vi "Actor Core.vi"(8 "error in":errorcluster, 11 "User Console":refnum<class "User Console.lvclass">) -> (0 "error out":errorcluster, 3 "Actor out":refnum<class "Actor.lvclass">)   [LabVIEW 2019, in "User Console Actor.lvlib" / "User Console.lvclass"]
doc: "This is Actor Core.vi, the main message handling loop for Actors. An actor usually just sits in this loop and processes messages as they arrive. Any error returned by the message Do.vi call will stop the loop, with error code 43 as the canonical signal to stop with no error sent to caller. Descendants may override that in Handle Error.vi."
uses:
  User Console.lvclass
  <vilib>/ActorFramework/Actor/Actor.lvclass
  <vilib>/ActorFramework/Stop Msg/Stop Msg.lvclass
  C:/Workspace/CLA/Elevator AF/Abstract User Console Actor/Abstract User Console Actor/Abstract User Console.lvclass
  C:/Program Files (x86)/National Instruments/LabVIEW 2019/vi.lib/ActorFramework/Actor/Actor.lvclass
  Abstract User Console Actor/Abstract User Console Actor/Abstract User Console.lvclass
  Elevator Controller Actor/Elevator Control Actor/States -Enum.ctl
  Elevator Controller Actor/Elevator Control Actor/Elevator Controller.lvclass
  Elevator Controller Actor/Elevator Controller Messages/Set State Msg/Set State Msg.lvclass
  Display Console/Display Console/Display Console.lvclass
  Door Buttons.ctl
  Elevator Call.ctl
  Floor Selection.ctl
panel:
  in  "Floor Selection":T1
  in  "Elevator Call":T2
  in  "Emergency Button":bool
  in  "Door Buttons":T3
  # "[Covers: UI1]"
  # "[Covers: UI2]"
  # "[Covers: UI2A] \n[Covers: UI2A1] \n[Covers: UI2A2]"
  # "[Covers: UI2B] \n[Covers: UI2B1] \n[Covers: UI2B2]"
  # "[Covers: UI2C] \n[Covers: UI2C1] \n[Covers: UI2C2] \n[Covers: UI2C3]"
  # "[Covers: UI2D] \n[Covers: UI2D1]"
  # "Fourth Floor"
  # "Third Floor"
  # "Second Floor"
  # "First Floor"
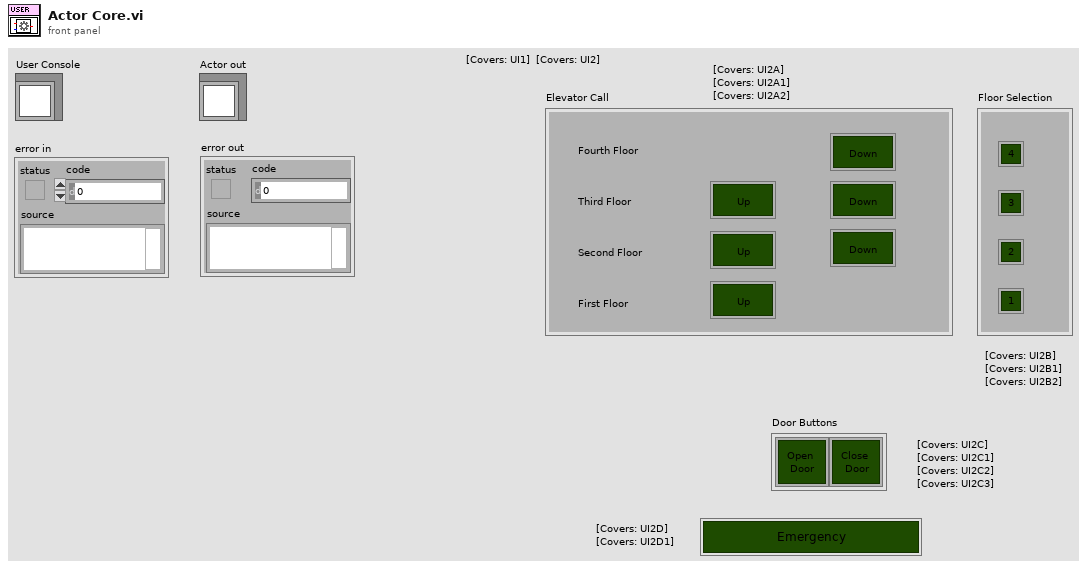
[diagram p1: front panel]
types:
  T1 = typedef "User Console Actor.lvlib/User Console.lvclass/Floor Selection.ctl" = cluster{"Floor4":bool, "Floor 3":bool, "Floor2":bool, "Floor1":bool}
  T2 = typedef "User Console Actor.lvlib/User Console.lvclass/Elevator Call.ctl" = cluster{"Up":bool, "Up 2":bool, "Up 3":bool, "Down":bool, "Down 2":bool, "Down 3":bool}
  T3 = typedef "User Console Actor.lvlib/User Console.lvclass/Door Buttons.ctl" = cluster{"Open Door":bool, "Close Door":bool}
  T4 = typedef "Elevator Controller Actor.lvlib/Elevator Controller.lvclass/States -Enum.ctl" = enum16{"Initial State", "Start and Move State", "Analysis State", "Continue Travel State", "Open and Close Door Sequence", "Stop at Floor", "No Request remaining", "Emergency Call", "Terminate Process"}
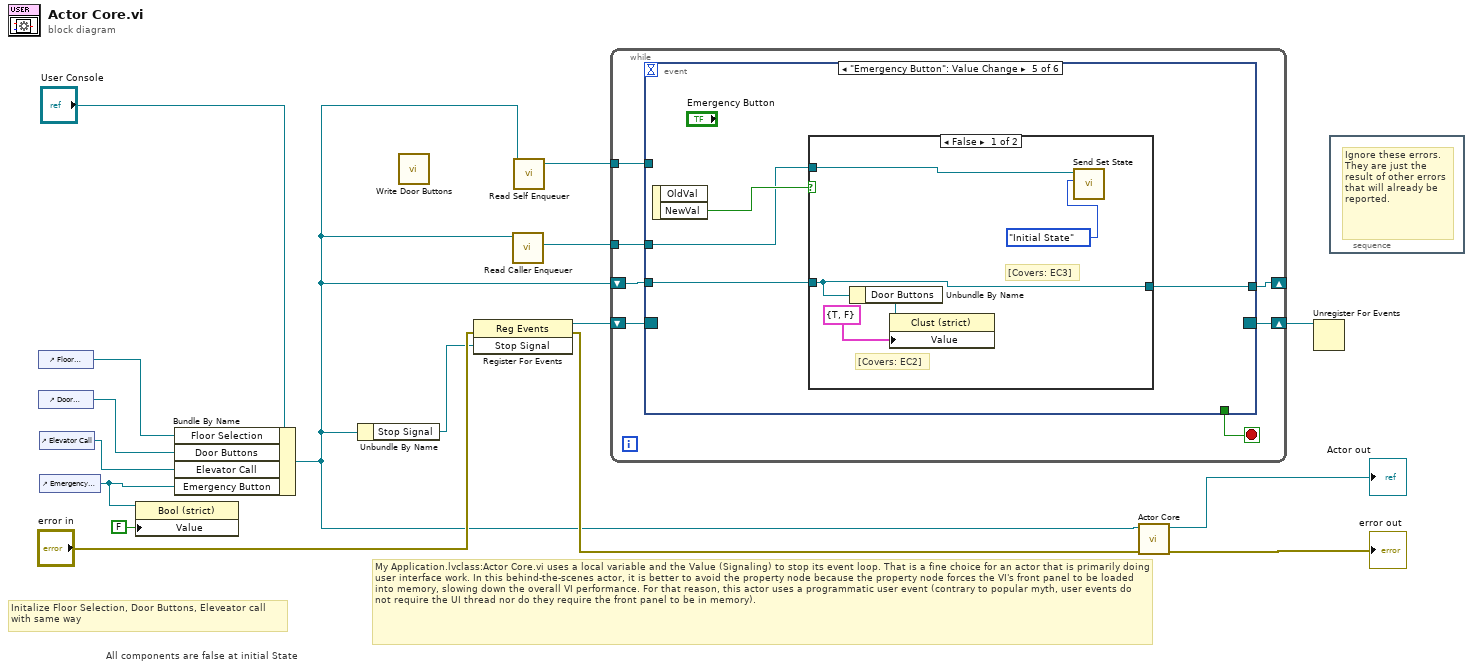
[diagram p0: block diagram]
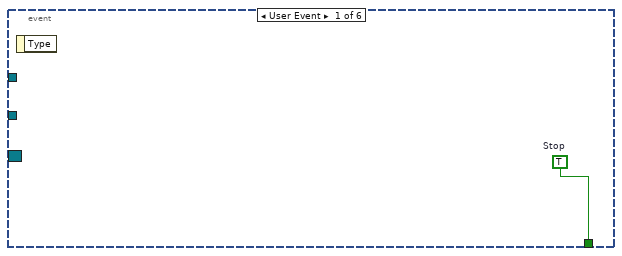
[diagram p2: hidden frame]
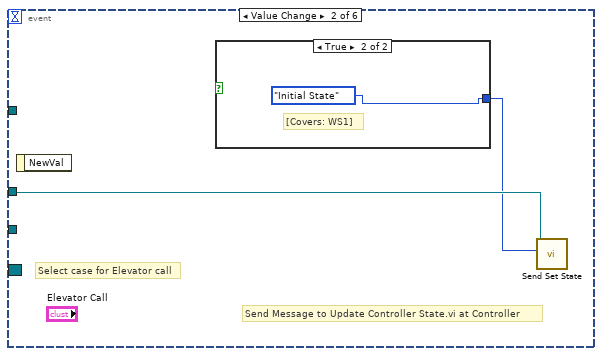
[diagram p3: hidden frame]
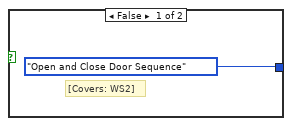
[diagram p4: hidden frame]
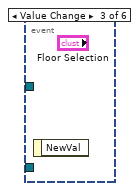
[diagram p5: hidden frame]
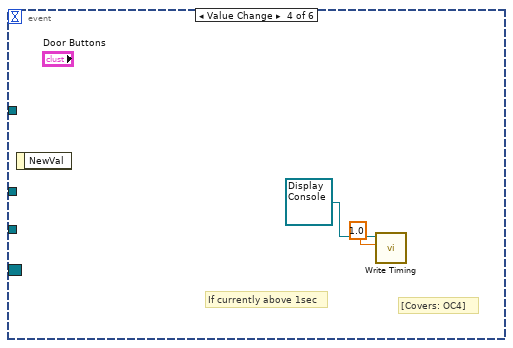
[diagram p6: hidden frame]
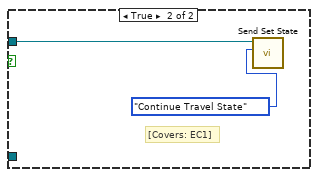
[diagram p7: hidden frame]
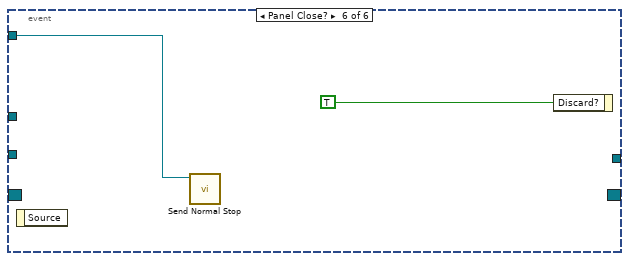
[diagram p8: hidden frame]
diagram:
  # "All components are false at initial State"
  # "Initalize Floor Selection, Door Buttons, Eleveator call \nwith same way"
  # "My Application.lvclass:Actor Core.vi uses a local variable and the Value (Signaling) to stop its event loop. That is a fine choice for an actor that is primarily doing user interface work. In this behind-the-scenes actor, it is better to avoid the property node because the property node forces the VI's front panel to be loaded into memory, slowing down the overall VI performance. For that reason, this actor uses a programmatic user event (contrary to popular myth, user events do not require the UI thread nor do they require the front panel to be in memory)."
  n1 = control-ref of="Floor Selection"() -> (w2:refnum<vi>)
  n2 = control-ref of="Door Buttons"() -> (w3:refnum<vi>)
  n3 = control-ref of="Elevator Call"() -> (w4:refnum<vi>)
  n4 = control-ref of="Emergency Button"() -> (w6:refnum<vi>)
  n5 = property class="Bool (strict)"(reference=w6, "Value"=FALSE) -> ()  [unwired: 1 in, 2 out]
  n6 = Bundle By Name(cluster="User Console", "Floor Selection"=w2, "Door Buttons"=w3, "Elevator Call"=w4, "Emergency Button"=w6) -> (w1:refnum<class "User Console.lvclass">)
  n7 = Unbundle By Name(w1) -> ("Stop Signal"=w8:refnum<user-event>)
  n8 = call-dynamic "Write Door Buttons.vi"() -> ()  [unwired: 10 in, 2 out]
  n9 = register-events(error in="error in", w8) -> (reference out=w13:refnum<event-registration>, error out=w11:errorcluster)  [unwired: 1 in]
  n10 = call <vilib>:"Read Caller Enqueuer.vi"("Actor"=w1) -> ("Caller Enqueuer"=w15:refnum<class "Message Enqueuer.lvclass">)  [unwired: 10 in]
  n11 = call <vilib>:"Read Self Enqueuer.vi"("Actor"=w1) -> ("Self Enqueuer"=w16:refnum<class "Message Enqueuer.lvclass">)  [unwired: 10 in]
  n12 = while {
    tunnel: w16 -> [w22]
    tunnel: w15 -> [w21]
    shift-right: [w19] -> w10
    shift-left: w13 -> [w20]
    shift-right: [w17] -> _
    shift-left: w1 -> [w18]
    stop <- w23 stop-if-true
    n13 = event shown="[4] \"Emergency Button\": Value Change" {
      selector: w20 -> [_ _ _ _ _ _]
      dyn-events: [_ _ _ _ _ _] -> w19
      timeout: _ -> [_ _ _ _ _ _]
      tunnel: [w24 _ _ _ _ _] -> w23
      tunnel: w22 -> [_ _ _ _ _ w43]
      tunnel: w21 -> [_ w26 _ _ w33 _]
      tunnel: w18 -> [_ _ _ _ w32 _]
      tunnel: [_ _ _ _ w31 _] -> w17
      event User Event {
        w24 = TRUE  # Stop
        n14 = event-data() -> ()  [unwired: 1 in, 1 out]
      }
      event Value Change {
        # "Select case for Elevator call"
        # "Send Message to Update Controller State.vi at Controller"
        n15 = event-data() -> ()  [unwired: 1 in, 1 out]
        n16 = case shown="\"Initial State\"" {
          selector: _ -> [_ _]
          tunnel: [States_-Enum."Open and Close Door Sequence" ("State") States_-Enum."Initial State" ("State")] -> w25
          frame False {
            # "[Covers: WS2]"
          }
          frame True {
            # "[Covers: WS1]"
          }
        }
        n17 = call "Send Set State.vi"("States"=w25, "Message Enqueuer"=w26) -> ()  [unwired: 8 in, 2 out]
      }
      event Value Change {
        n18 = event-data() -> ()  [unwired: 1 in, 1 out]
      }
      event Value Change {
        # "If currently above 1sec"
        # "[Covers: OC4]"
        n19 = event-data() -> ()  [unwired: 1 in, 1 out]
        n20 = call-dynamic "Write Timing.vi"("timing"=1.0, "Display Console in"=refnum<class "Display Console.lvclass"> refnum ("Display Console Actor.lvlib:Display Console.lvclass")) -> ()  [unwired: 8 in, 2 out]
      }
      event "Emergency Button": Value Change {
        n21 = event-data() -> ("NewVal"=w34:bool)  [unwired: 1 in, 1 out]
        n22 = case shown="False" w34 {
          tunnel: w33 -> [w38 w40]
          tunnel: w32 -> [w35 _]
          tunnel: [w35 _] -> w31
          frame False {
            # "[Covers: EC2]"
            # "[Covers: EC3]"
            n23 = Unbundle By Name(w35) -> ("Door Buttons"=w37:refnum<vi>)
            n24 = property class="Clust (strict)"(reference=w37, "Value"=T3 {"Open Door"=TRUE, "Close Door"=FALSE} ("Door Buttons")) -> ()  [unwired: 1 in, 2 out]
            n25 = call "Send Set State.vi"("States"=States_-Enum."Initial State" ("State"), "Message Enqueuer"=w38) -> ()  [unwired: 8 in, 2 out]
          }
          frame True {
            # "[Covers: EC1]"
            n26 = call "Send Set State.vi"("States"=States_-Enum."Continue Travel State" ("State"), "Message Enqueuer"=w40) -> ()  [unwired: 8 in, 2 out]
          }
        }
      }
      event Panel Close? {
        n27 = event-data() -> ()  [unwired: 1 in, 1 out]
        n28 = call <vilib>:"Send Normal Stop.vi"("Message Enqueuer"=w43) -> ()  [unwired: 10 in, 1 out]
        n29 = event-data("Discard?"=TRUE) -> ()  [unwired: 1 in, 1 out]
      }
    }
  }
  n30 = call-parent "Actor Core.vi"("error in"=w11, "Actor in"=w1) -> ("error out"=→"error out":errorcluster, "Actor out"=→"Actor out":refnum<class "Actor.lvclass">)  [unwired: 8 in]
  n31 = Unregister For Events(event registration refnum=w10) -> ()  [unwired: 1 in, 1 out]
  n32 = stacked-sequence {
    frame #0 {
      # "Ignore these errors.\nThey are just the result of other errors that will already be reported."
    }
  }
